vi "4 memory dds 8SPC.vi"(8 "referenses":T1={"clock x2"="IO Socket\\Data Clock 2x", "Memory In"="pulse on memory", "Memory In 2"="pulse on memory", "Memory In 3"="pulse on memory", "Memory In 4"="pulse on memory"}, 9 "pdw in":T3 {"frequency shift" format="%#_12f"}, 10 "free DDS before me?":bool, 11 "new PDW in":bool) -> (0 "output valid":bool, 1 "state of every DDS":bool[](array[boolean]), 2 "have free DDS":bool, 3 "IQ out":T2[](array[typedef]))   [LabVIEW 2021]
doc: "transmit pulse with one free DDS inside.\nmust have no DDS before him (the distribute is to give the lowest mun DDS the pulse)"
uses:
  pulse_tx_vis/pdw.ctl
  pulse_tx_vis/CTL/mode_type.ctl
  <instrlib>/_niInstr/DSP/v1/Shared/Public/IQ Data.ctl
  <instrlib>/_niInstr/DSP/v1/Shared/niInstr DSP v1 Shared.lvlib
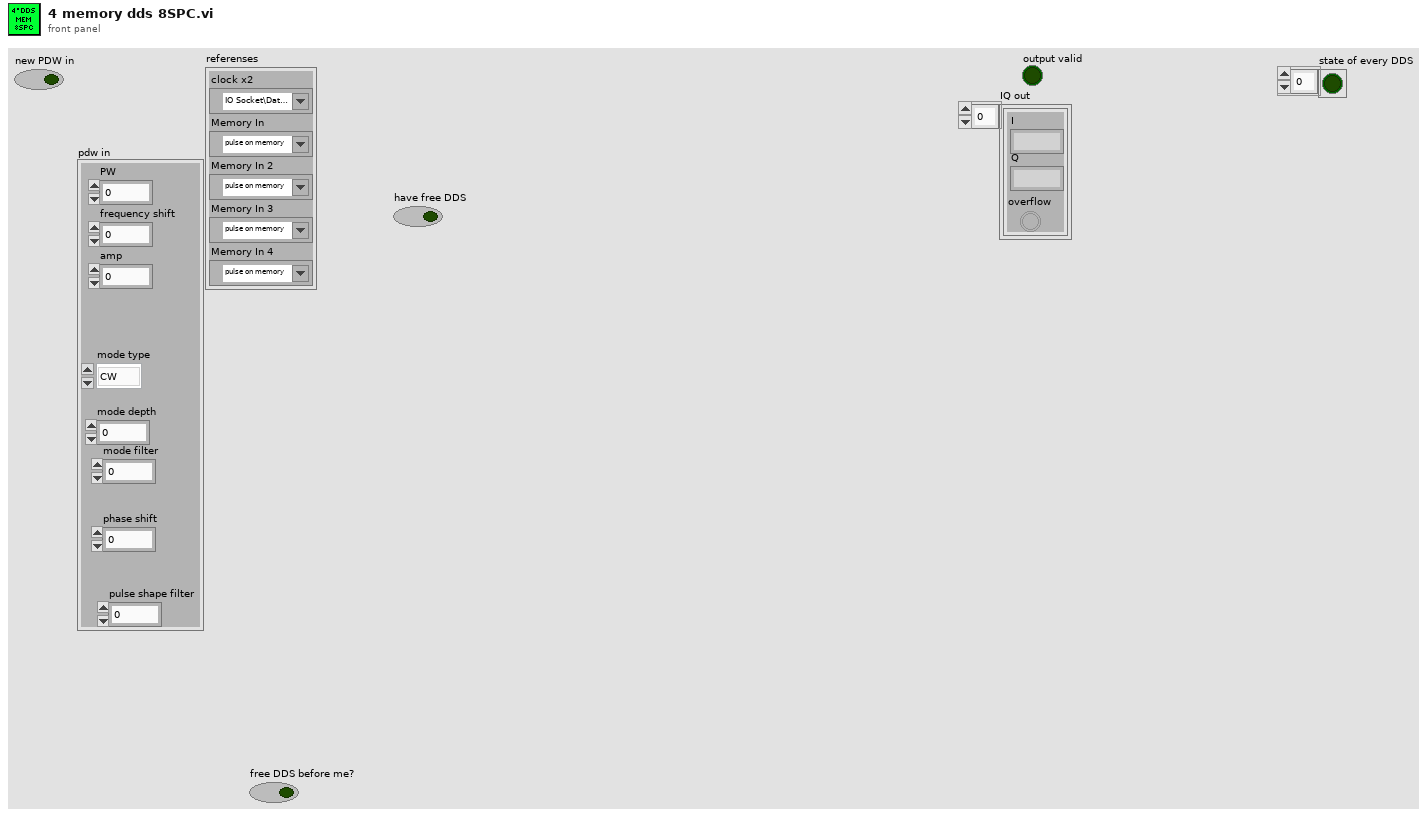
[diagram p1: front panel]
types:
  T1 = cluster{"clock x2":refnum<k21>, "Memory In":refnum<k21>, "Memory In 2":refnum<k21>, "Memory In 3":refnum<k21>, "Memory In 4":refnum<k21>}
  T2 = typedef "niInstr DSP v1 Shared.lvlib/IQ Data.ctl" = cluster{"I":fxp<+/-,18,1>, "Q":fxp<+/-,18,1>, "overflow":bool}
  T3 = typedef "pdw.ctl" = cluster{"PW":u32, "frequency shift":fxp<+/-,48,0>, "amp":fxp<+/-,18,1>, "mode type":T4, "mode depth":u32, "mode filter":u8, "phase shift":fxp<+/-,16,1>, "pulse shape filter":u8}
  T4 = typedef "mode_type.ctl" = enum8{"CW", "from memory 1", "NC - cw", "LFM", "BPSK", "QPSK"}
  T5 = cluster{"clock x2":refnum<k21>, "Memory In":refnum<k21>}
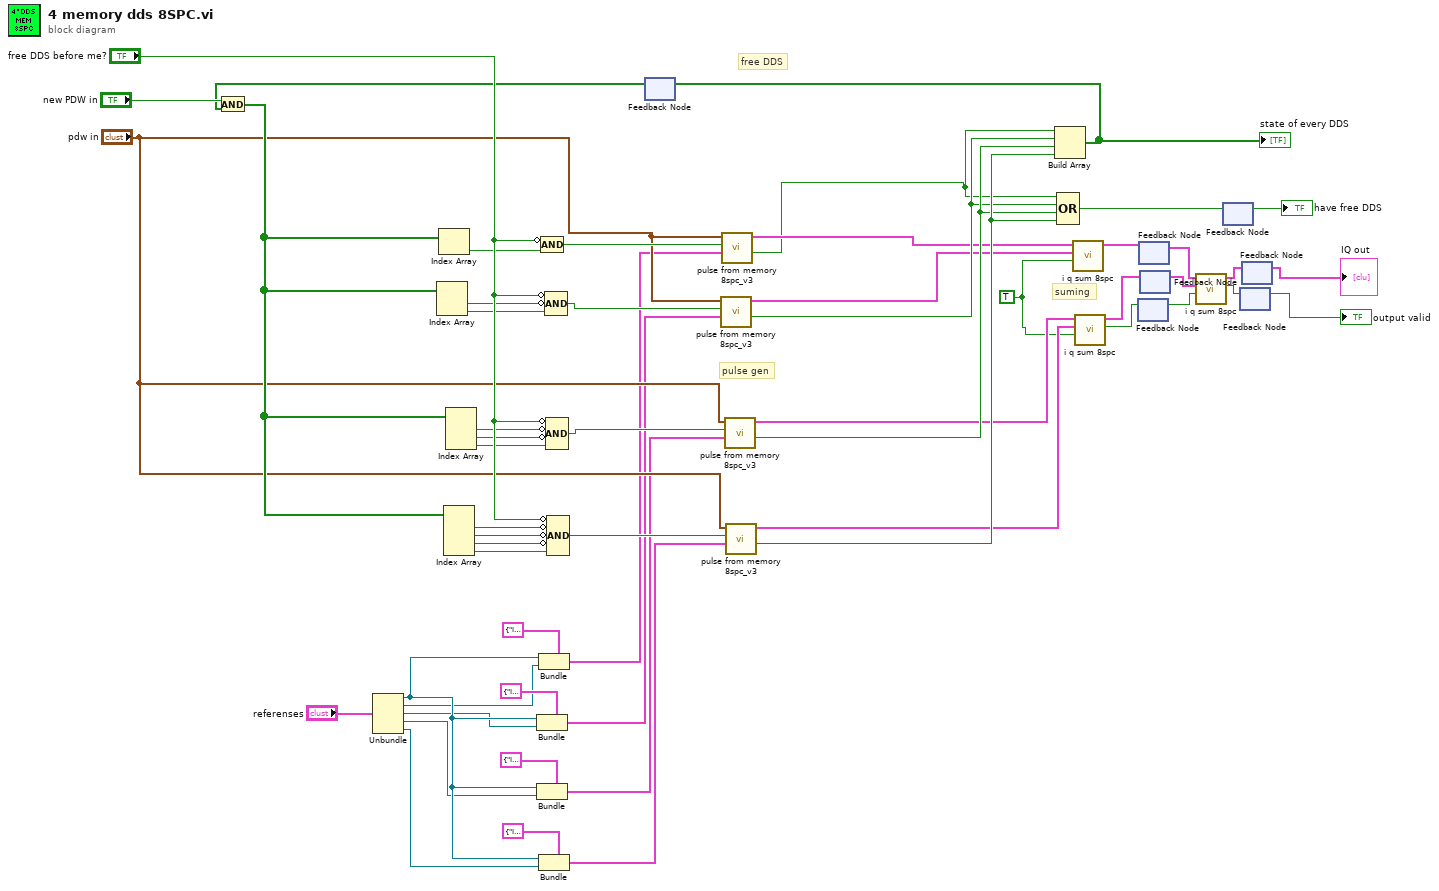
[diagram p0: block diagram]
diagram:
  w15 = TRUE ("input valid")
  # "free DDS"
  # "suming"
  # "pulse gen"
  n1 = Unbundle("referenses") -> ("clock x2"=w9:refnum<k21>, "Memory In"=w5:refnum<k21>, "Memory In 2"=w6:refnum<k21>, "Memory In 3"=w7:refnum<k21>, "Memory In 4"=w8:refnum<k21>)
  n2 = Bundle(cluster=T5 {"clock x2"="IO Socket\\Data Clock 2x", "Memory In"="pulse on memory"} ("referenses"), "clock x2"=w9, "Memory In"=w6) -> (w3:T5)
  n3 = Bundle(cluster=T5 {"clock x2"="IO Socket\\Data Clock 2x", "Memory In"="pulse on memory"} ("referenses"), "clock x2"=w9, "Memory In"=w7) -> (w2:T5)
  n4 = Bundle(cluster=T5 {"clock x2"="IO Socket\\Data Clock 2x", "Memory In"="pulse on memory"} ("referenses"), "clock x2"=w9, "Memory In"=w5) -> (w4:T5)
  n5 = Bundle(cluster=T5 {"clock x2"="IO Socket\\Data Clock 2x", "Memory In"="pulse on memory"} ("referenses"), "clock x2"=w9, "Memory In"=w8) -> (w1:T5)
  n6 = feedback #1() -> (w31:bool[])  [unwired: 1 in]
  n7 = And(x="new PDW in", y=w31) -> (x .and. y?=w30:bool[])
  n8 = Index Array(array=w30) -> (element #1=w42:bool, element #2=w40:bool)  [unwired: 2 in]
  n9 = Index Array(array=w30) -> (element=w38:bool)  [unwired: 1 in]
  n10 = Index Array(array=w30) -> (element #1=w50:bool, element #2=w49:bool, element #3=w48:bool, element #4=w47:bool)  [unwired: 4 in]
  n11 = Index Array(array=w30) -> (element #1=w46:bool, element #2=w45:bool, element #3=w44:bool)  [unwired: 3 in]
  n12 = Compound Arithmetic op=AND(invert "free DDS before me?", w38) -> (w39:bool)
  n13 = Compound Arithmetic op=AND(invert "free DDS before me?", invert w42, w40) -> (w41:bool)
  n14 = Compound Arithmetic op=AND(invert "free DDS before me?", invert w46, invert w45, w44) -> (w43:bool)
  n15 = Compound Arithmetic op=AND(invert "free DDS before me?", invert w50, invert w49, invert w48, w47) -> (w51:bool)
  n16 = call "pulse from memory 8spc_v3.vi"("referenses"=w3, "start this pulse"=w41, "PDW"="pdw in") -> ("free DDS"=w52:bool, "IQ_out"=w35:T2[])  [unwired: 7 in]
  n17 = call "pulse from memory 8spc_v3.vi"("referenses"=w4, "start this pulse"=w39, "PDW"="pdw in") -> ("free DDS"=w16:bool, "IQ_out"=w34:T2[])  [unwired: 7 in]
  n18 = call "pulse from memory 8spc_v3.vi"("referenses"=w2, "start this pulse"=w43, "PDW"="pdw in") -> ("free DDS"=w53:bool, "IQ_out"=w36:T2[])  [unwired: 7 in]
  n19 = call "pulse from memory 8spc_v3.vi"("referenses"=w1, "start this pulse"=w51, "PDW"="pdw in") -> ("free DDS"=w54:bool, "IQ_out"=w37:T2[])  [unwired: 7 in]
  n20 = Build Array(w16, w52, w53, w54) -> (w33:bool[])
  "state of every DDS" <- w33
  n21 = feedback-in #1(w33) -> ()
  n22 = Compound Arithmetic op=OR(w16, w52, w53, w54) -> (w29:bool)
  n23 = call "i q sum 8spc.vi"("input valid"=w15, "IQ in 2"=w35, "IQ in"=w34) -> ("IQ out"=w26:T2[])  [unwired: 7 in, 1 out]
  n24 = call "i q sum 8spc.vi"("input valid"=w15, "IQ in 2"=w37, "IQ in"=w36) -> ("output valid"=w24:bool, "IQ out"=w25:T2[])  [unwired: 7 in]
  n25 = feedback-in #2(w24) -> ()
  n26 = feedback #2() -> (w23:bool)  [unwired: 1 in]
  n27 = feedback #3() -> (w21:T2[])  [unwired: 1 in]
  n28 = feedback-in #3(w26) -> ()
  n29 = feedback #4() -> (w22:T2[])  [unwired: 1 in]
  n30 = feedback-in #4(w25) -> ()
  n31 = call "i q sum 8spc.vi"("input valid"=w23, "IQ in 2"=w22, "IQ in"=w21) -> ("output valid"=w18:bool, "IQ out"=w20:T2[])  [unwired: 7 in]
  n32 = feedback #5() -> (→"have free DDS":bool)  [unwired: 1 in]
  n33 = feedback-in #5(w29) -> ()
  n34 = feedback #6() -> (→"output valid":bool)  [unwired: 1 in]
  n35 = feedback-in #6(w18) -> ()
  n36 = feedback #7() -> (→"IQ out":T2[])  [unwired: 1 in]
  n37 = feedback-in #7(w20) -> ()
